vi "PH_Beckhoff_Application.declare digital PILS internal InputTags.vi"() -> (0 "Digital Inputs":T2, 1 "Description":string)   [LabVIEW 2014, in "PH_Beckhoff_Application.lvlib"]
uses:
  PH_Beckhoff_Application.lvlib
  PH_Beckhoff/PH_Beckhoff.Digital Inputs.ctl
  PH_Beckhoff/PH_Beckhoff.lvlib
panel:
  in  "Digital Input Value":T1
  out "Right Size?":bool
  # "Let this VI run to check the size!"
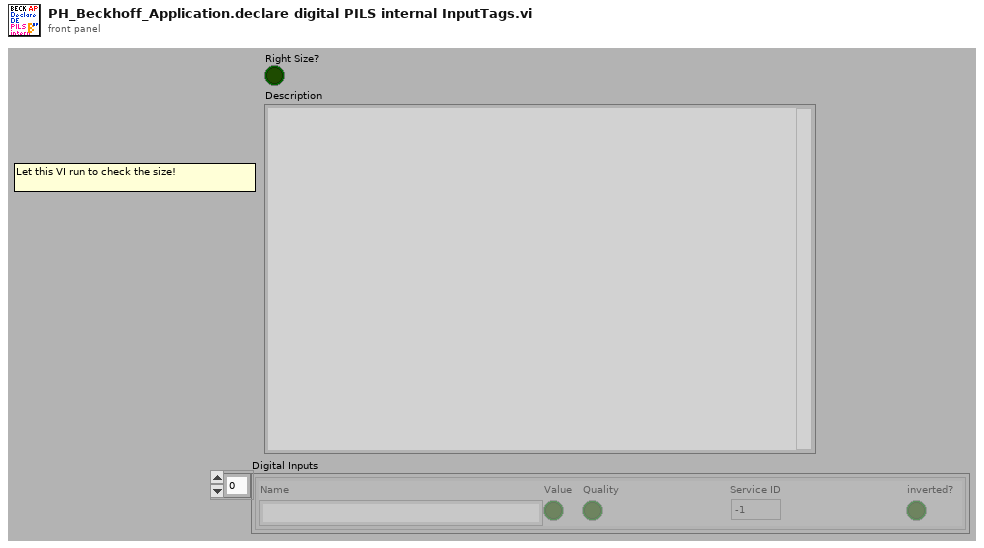
[diagram p1: front panel]
types:
  T1 = cluster{"Name":string, "Value":bool, "Quality":bool, "Service ID":i32, "inverted?":bool}
  T2 = typedef "PH_Beckhoff.lvlib/PH_Beckhoff.Digital Inputs.ctl" = cluster{"Name":string, "Value":bool, "Quality":bool, "Service ID":i32, "inverted?":bool}[]
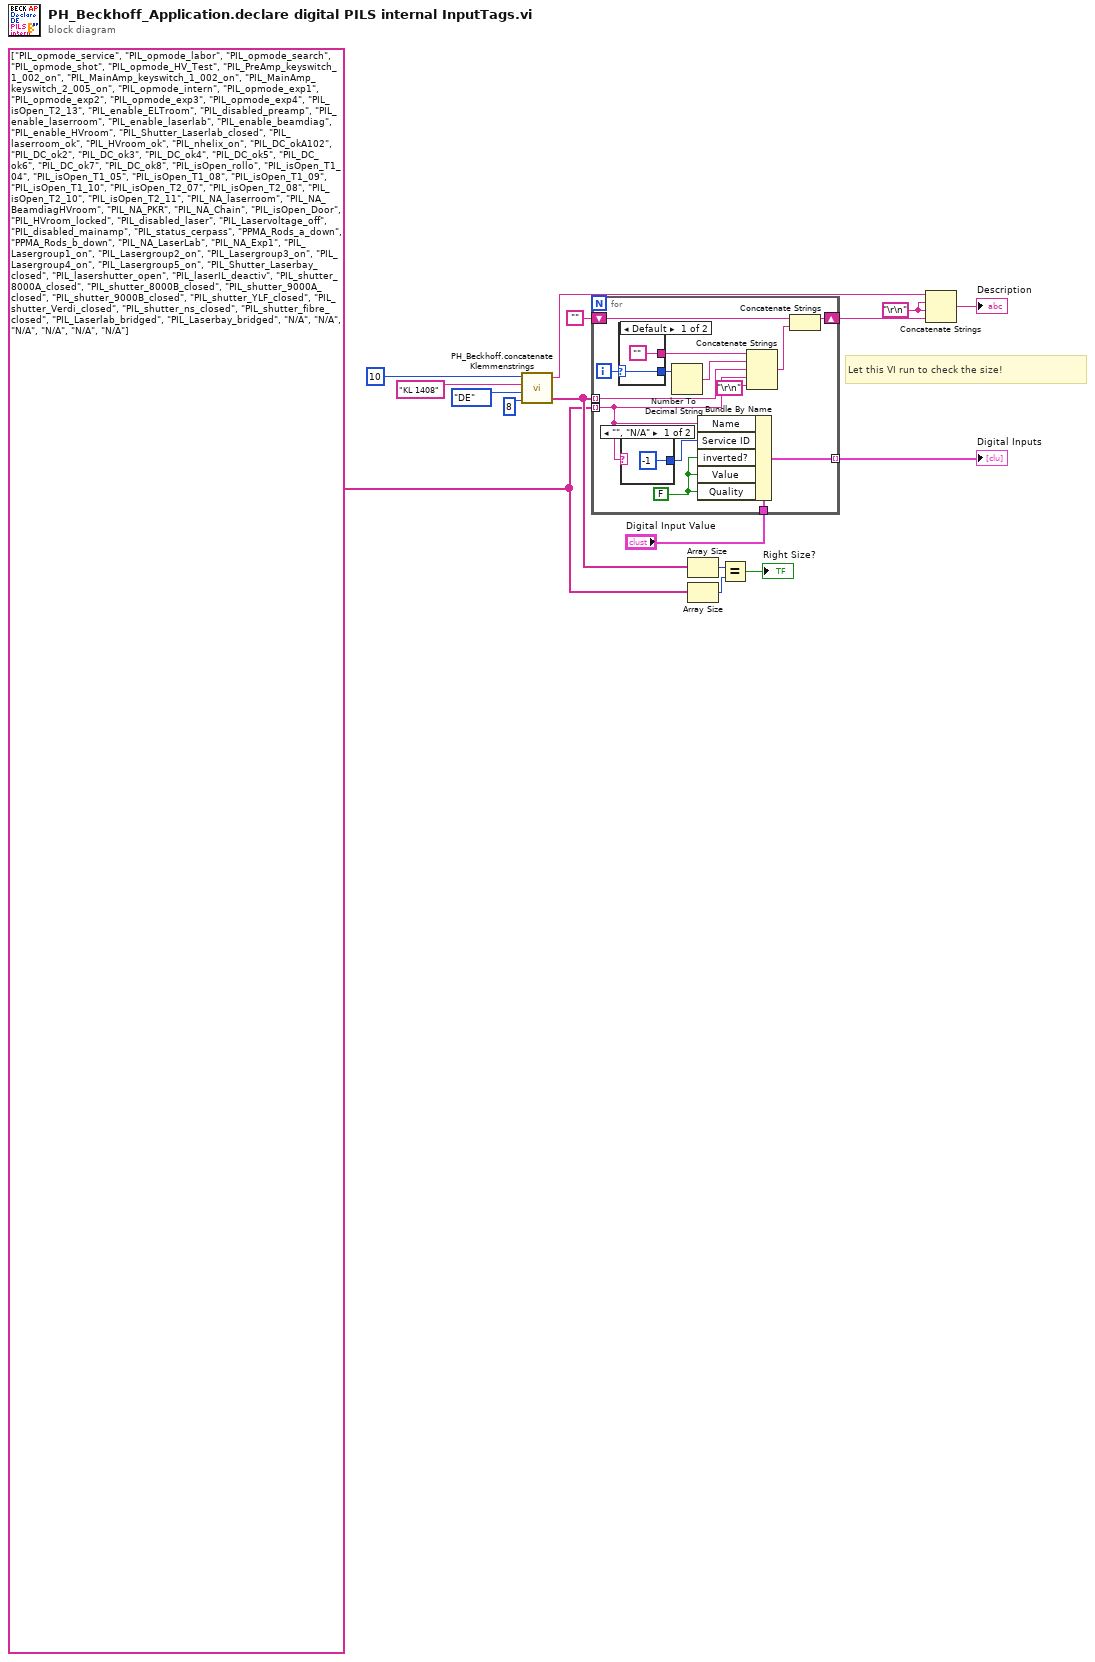
[diagram p0: block diagram]
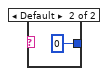
[diagram p2: hidden frame]
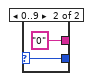
[diagram p3: hidden frame]
diagram:
  w1 = string[] ["PIL_opmode_service", "PIL_opmode_labor", "PIL_opmode_search", "PIL_opmode_shot", "PIL_opmode_HV_Test", "PIL_PreAmp_keyswitch_1_002_on", "PIL_MainAmp_keyswitch_1_002_on", "PIL_MainAmp_keyswitch_2_005_on", "PIL_opmode_intern", "PIL_opmode_exp1", "PIL_opmode_exp2", "PIL_opmode_exp3", "PIL_opmode_exp4", "PIL_isOpen_T2_13", "PIL_enable_ELTroom", "PIL_disabled_preamp", "PIL_enable_laserroom", "PIL_enable_laserlab", "PIL_enable_beamdiag", "PIL_enable_HVroom", "PIL_Shutter_Laserlab_closed", "PIL_laserroom_ok", "PIL_HVroom_ok", "PIL_nhelix_on", "PIL_DC_okA102", "PIL_DC_ok2", "PIL_DC_ok3", "PIL_DC_ok4", "PIL_DC_ok5", "PIL_DC_ok6", "PIL_DC_ok7", "PIL_DC_ok8", "PIL_isOpen_rollo", "PIL_isOpen_T1_04", "PIL_isOpen_T1_05", "PIL_isOpen_T1_08", "PIL_isOpen_T1_09", "PIL_isOpen_T1_10", "PIL_isOpen_T2_07", "PIL_isOpen_T2_08", "PIL_isOpen_T2_10", "PIL_isOpen_T2_11", "PIL_NA_laserroom", "PIL_NA_BeamdiagHVroom", "PIL_NA_PKR", "PIL_NA_Chain", "PIL_isOpen_Door", "PIL_HVroom_locked", "PIL_disabled_laser", "PIL_Laservoltage_off", "PIL_disabled_mainamp", "PIL_status_cerpass", "PPMA_Rods_a_down", "PPMA_Rods_b_down", "PIL_NA_LaserLab", "PIL_NA_Exp1", "PIL_Lasergroup1_on", "PIL_Lasergroup2_on", "PIL_Lasergroup3_on", "PIL_Lasergroup4_on", "PIL_Lasergroup5_on", "PIL_Shutter_Laserbay_closed", "PIL_lasershutter_open", "PIL_laserIL_deactiv", "PIL_shutter_8000A_closed", "PIL_shutter_8000B_closed", "PIL_shutter_9000A_closed", "PIL_shutter_9000B_closed", "PIL_shutter_YLF_closed", "PIL_shutter_Verdi_closed", "PIL_shutter_ns_closed", "PIL_shutter_fibre_closed", "PIL_Laserlab_bridged", "PIL_Laserbay_bridged", "N/A", "N/A", "N/A", "N/A", "N/A", "N/A"] ("Array")
  w12 = "\r\n"
  # "Let this VI run to check the size!"
  n1 = call "PH_Beckhoff.concatenate Klemmenstrings.vi"("# of In- or Outputs"=8, "Type"=enum16{"AE", "AA", "DE", "DA"}."DE", "Klemmenname"="KL 1408", "Quantity"=10 ("size(s)")) -> ("concatenated string array"=w7:string[], "\"<Type>: <Quantity> x <Klemmenname>\""=w9:string)  [unwired: 1 out]
  n2 = for {
    tunnel: w1 -> [w21] mode=indexing
    tunnel: w7 -> [w26] mode=indexing
    shift-right: [w24] -> w13
    shift-left: "" -> [w23]
    tunnel: "Digital Input Value" -> [w22]
    tunnel: [w19] -> w2 mode=indexing
    i -> [w30]
    w18 = FALSE ("Quality")
    n3 = case shown="Default" w30 {
      selector: w30 -> [w33 w36]
      tunnel: [w33 w36] -> w29
      tunnel: ["" "0"] -> w28
      frame Default {
      }
      frame 0..9 {
      }
    }
    n4 = case shown="\"\", \"N/A\"" w21 {
      tunnel: [-1 0] -> w20
      frame "", "N/A" {
      }
      frame Default {
      }
    }
    n5 = Number To Decimal String(number=w29) -> (decimal integer string=w27:string)  [unwired: 1 in]
    n6 = Bundle By Name(cluster=w22, "Name"=w21, "Service ID"=w20, "inverted?"=w18, "Value"=w18, "Quality"=w18) -> (w19:T1)
    n7 = Concatenate Strings(w28, w27, w26, w21, "\r\n") -> (w25:string)
    n8 = Concatenate Strings(w23, w25) -> (w24:string)
  }
  "Digital Inputs" <- w2
  n9 = Array Size(array=w7) -> (size(s)=w6:i32)
  n10 = Array Size(array=w1) -> (size(s)=w4:i32)
  n11 = Equal?(x=w6, y=w4) -> (x = y?=→"Right Size?":bool)
  n12 = Concatenate Strings(w9, w12, w12, w13) -> (→"Description":string)
